vi "Test_WriteValue_ReadValue_ValueReturned.vi"(8 "error in (no error)":errorcluster, 11 "TestCase in":refnum<class "TestEventTransport.lvclass">) -> (0 "error out":errorcluster, 3 "TestCase out":refnum<class "TestEventTransport.lvclass">)   [LabVIEW 2017, in "TestEventTransport.lvclass"]
uses:
  TestEventTransport.lvclass
  Source/Concrete/EventTransport/EventTransport.lvclass/EventTransport.ctl
  Source/Concrete/EventTransport/EventTransport.lvclass
  C:/Git/composed-transport/Source/ITransport/ITransport.lvclass
  Source/ITransport/ITransport.lvclass
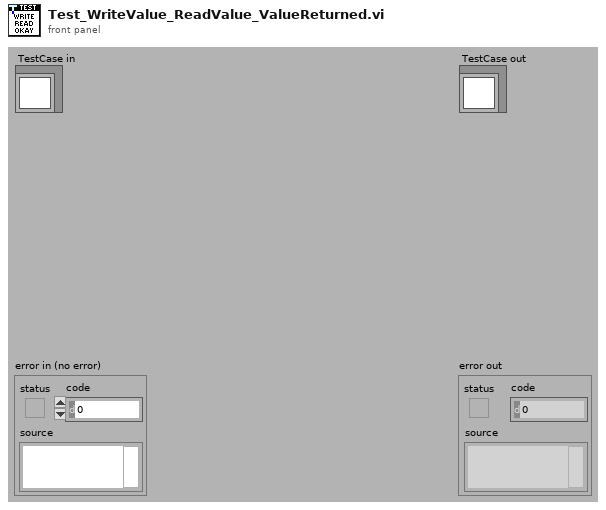
[diagram p1: front panel]
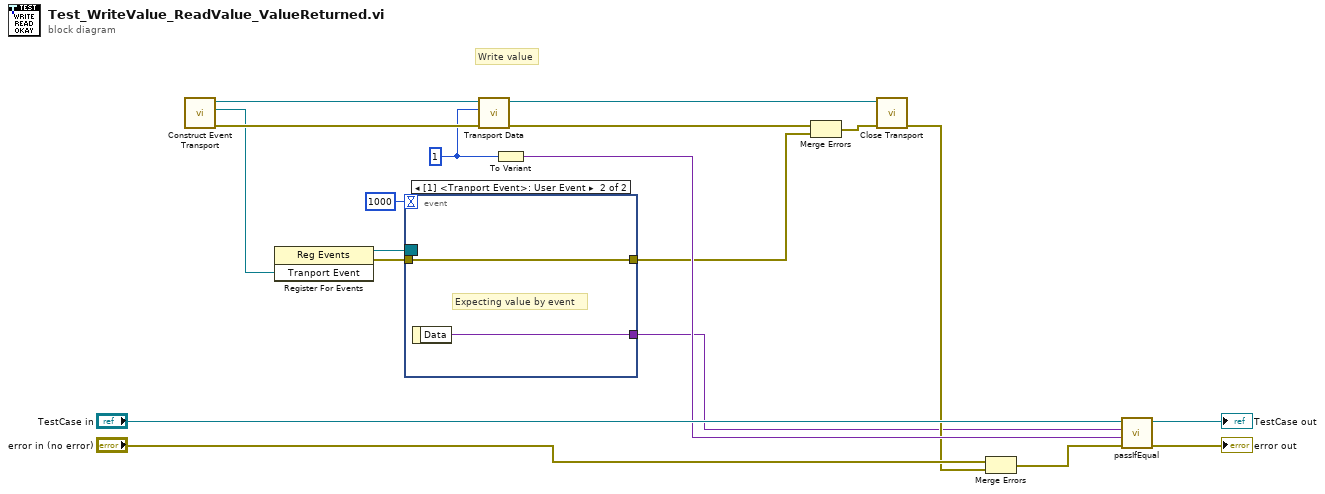
[diagram p0: block diagram]
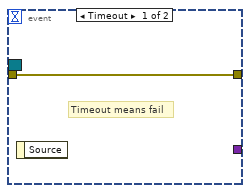
[diagram p2: hidden frame]
diagram:
  w12 = 1
  # "Write value"
  n1 = call "Construct Event Transport.vi"() -> ("error out"=w13:errorcluster, "Tranport Event"=w6:refnum<user-event>, "EventTransport"=w15:refnum<class "EventTransport.lvclass">)  [unwired: 9 in]
  n2 = register-events(w6) -> (reference out=w7:refnum<event-registration>, error out=w3:errorcluster)  [unwired: 2 in]
  n3 = event shown="[1] <Tranport Event>: User Event" {
    selector: w7 -> [_ _]
    dyn-events: _ -> [_ _]
    timeout: 1000 -> [_ _]
    tunnel: [_ w22] -> w5
    tunnel: w3 -> [w20 w21]
    tunnel: [w20 w21] -> w1
    event Timeout {
      # "Timeout means fail"
      n4 = event-data() -> ()  [unwired: 1 in, 1 out]
    }
    event User Event {
      # "Expecting value by event"
      n5 = event-data() -> ("Data"=w22:variant)  [unwired: 1 in]
    }
  }
  n6 = call "Transport Data.vi"("error in (no error)"=w13, "Value"=w12, "ITransport in"=w15) -> ("error out"=w8:errorcluster, "ITransport out"=w10:refnum<class "EventTransport.lvclass">)  [unwired: 7 in]
  n7 = To Variant(anything=w12) -> (Variant=w11:variant)
  n8 = Merge Errors(w8, w1) -> (w2:errorcluster)
  n9 = call-dynamic "Close Transport.vi"("error in (no error)"=w2, "EventTransport"=w10) -> ("error out"=w9:errorcluster)  [unwired: 9 in]
  n10 = Merge Errors("error in (no error)", w9) -> (w14:errorcluster)
  n11 = call-dynamic "passIfEqual.vi"("error in (no error)"=w14, "y"=w11, "x"=w5, "TestCase in"="TestCase in") -> ("error out"=→"error out":errorcluster, "TestCase out"=→"TestCase out":refnum<class "TestEventTransport.lvclass">)  [unwired: 6 in]
